vi "Daten Serialisieren - 64xbool.vi"(9 "Frame-ID":u32, 10 "Aktuelle Zeit":timestamp, 11 "Fehler":u64) -> (0 "Frame-ID letzter Wert":u32, 2 "data":T1[](array[typedef])=[{"timestamp"=timestamp(0 s since 1904-01-01), "payload"=[0, 2, 3, 4, 5, 6, 7, 8], "identifier"=2, "type"=0, "extended?"=FALSE, "echo?"=FALSE}, {"timestamp"=timestamp(0 s since 1904-01-01), "payload"=[0, 1, 2, 3, 4, 5, 6, 7], "identifier"=3, "type"=0, "extended?"=FALSE, "echo?"=FALSE}] {"payload" format="%x"; "timestamp" format="%<%.7X\n%x>T"; "type" items=["CAN Data"=0, "CAN Remote"=1, "CAN Bus Error"=2, "CAN 2.0 Data"=8, "CAN FD Data"=16, "CAN FD+BRS Data"=24, "J1939 Data"=192, "Delay"=224, "Log Trigger"=225, "Start Trigger"=226]; "identifier" format="%x"})   [LabVIEW 2020, in "CAN Interface.lvlib"]
uses:
  CAN Interface.lvlib
  <vilib>/xnet/xnet.llb/XNET Frame CAN.ctl
  <vilib>/xnet/xnet.llb/XNET Frame Type CAN.ctl
panel:
  out "Numerisch":i32
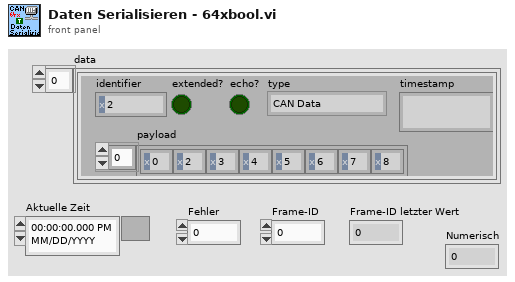
[diagram p1: front panel]
types:
  T1 = typedef "XNET Frame CAN.ctl" = cluster{"timestamp":timestamp, "payload":u8[], "identifier":u32, "type":T2, "extended?":bool, "echo?":bool}
  T2 = typedef "XNET Frame Type CAN.ctl" = u8
  T3 = enum16{"big-endian, network order", "native, host order", "little-endian"}
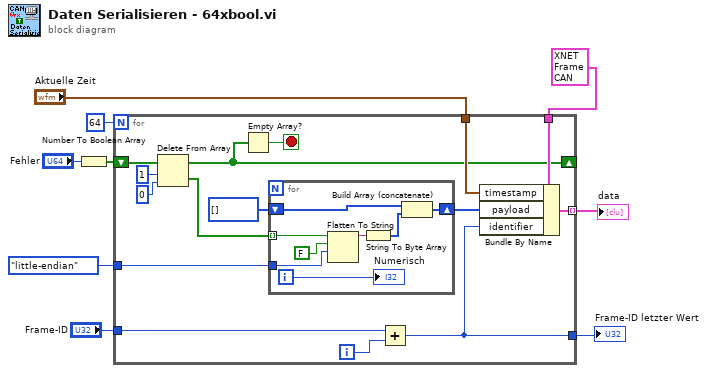
[diagram p0: block diagram]
diagram:
  n1 = Number To Boolean Array(number="Fehler") -> (Boolean array=w2:bool[])
  n2 = for {
    N: 64 -> [_]
    tunnel: T1 {"timestamp"=timestamp(0 s since 1904-01-01), "payload"=[0, 2, 3, 4, 5, 6, 7, 8], "identifier"=2, "type"=0, "extended?"=FALSE, "echo?"=FALSE} ("CAN frame") -> [w24]
    tunnel: "Frame-ID" -> [w22]
    tunnel: "Aktuelle Zeit" -> [w21]
    tunnel: [w20] -> w6 mode=indexing
    shift-right: [w16] -> _
    shift-left: w2 -> [w19]
    tunnel: [w11] -> w7
    tunnel: T3."little-endian" ("Byte-Reihenfolge (0:Big-Endian, Netzwerkreihenfolge)") -> [w10]
    i -> [w23]
    stop <- w15 stop-if-true
    n3 = Delete From Array(array=w19, length=1 ("Länge"), index=0 ("Index")) -> (deleted portion=w14:bool[], array with subset deleted=w16:bool[])
    n4 = Empty Array?(array=w16) -> (empty?=w15:bool)
    n5 = for {
      tunnel: w14 -> [w26] mode=indexing
      shift-right: [w28] -> w12
      shift-left: u8[] [] ("Vorzeichenloses Byte-Array") -> [w29]
      tunnel: w10 -> [w25]
      i -> [w27]
      n6 = Flatten To String(anything=w26, prepend array or string size? (T)=FALSE ("Array- oder String-Größe voranstellen? (T)"), byte order (0:big-endian, network order)=w25) -> (data string=w32:string)  [unwired: 1 in, 2 out]
      n7 = String To Byte Array(string=w32) -> (unsigned byte array=w30:u8[])
      n8 = Build Array (concatenate)(w29, w30) -> (w28:u8[])
      "Numerisch" <- w27
    }
    n9 = Add(x=w22, y=w23) -> (x+y=w11:u32)
    n10 = Bundle By Name(cluster=w24, "timestamp"=w21, "payload"=w12, "identifier"=w11) -> (w20:T1)
  }
  "data" <- w6
  "Frame-ID letzter Wert" <- w7
